vi "AutonIndexSave.vi"(1 "index":i32) -> ()   [LabVIEW 2013]
uses:
  <vilib>/Utility/config.llb/Write Key (I32).vi
  <vilib>/Utility/config.llb/NI_LVConfig.lvlib
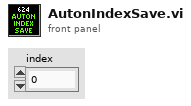
[diagram p1: front panel]
types:
  T1 = typedef "NI_LVConfig.lvlib/Config Data RefNum.ctl" = refnum<k1>
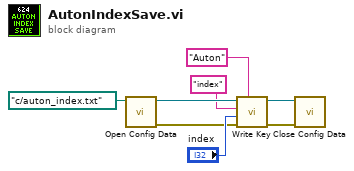
[diagram p0: block diagram]
diagram:
  n1 = call <vilib>:"Open Config Data.vi"("configuration file path"=path "c:/auton_index.txt") -> ("error out"=w1:errorcluster, "refnum"=w7:T1)  [unwired: 8 in, 1 out]
  n2 = call-poly <vilib>:"Write Key.vi"("section"="Auton", "error in (no error)"=w1, "value"="index", "key"="index", "refnum"=w7) -> ("error out"=w3:errorcluster, "refnum out"=w2:T1)  [unwired: 4 in, 1 out]
  n3 = call <vilib>:"Close Config Data.vi"("error in (no error)"=w3, "refnum"=w2) -> ()  [unwired: 8 in, 2 out]
